vi "Create Scalars for Numeric.vi"() -> ()   [LabVIEW 2021, in "EDT VI Script.lvlib"]
uses:
  Numeric Representation to Type Cast.ctl
  <vilib>/numeric/LVNumericRepresentation.ctl
  EDT VI Script.lvlib
panel:
  in  "Template VI Path":path=path "C:/Users/OneEd/OneDrive/Documents/LabVIEW/edt.lib/numeric.lib/Random in Range (Double).vi"
  in  "PlaceHolders":string[](array[string])=["hi", "lo", "random"]
  out "Slide":dbl(slide) scale=0.0..1.0
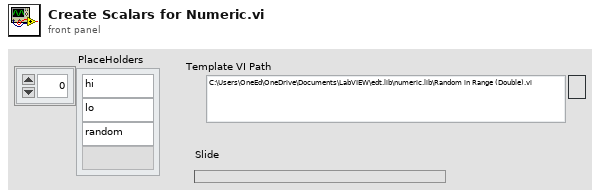
[diagram p1: front panel]
types:
  T1 = typedef "EDT VI Script.lvlib/Numeric Representation to Type Cast.ctl" = map{T2, i32}
  T2 = typedef "LVNumericRepresentation.ctl" = enum32{"Extended Precision", "Double Precision", "Single Precision", "Long", "Word", "Byte", "Unsigned Long", "Unsigned Word", "Unsigned Byte", "Complex Extended", "Complex Double", "Complex Single", "Quad", "Unsigned Quad", "Fixed-Point"}
  T3 = cluster{"Placeholder Name":string, "Function Type":i32}
  T4 = cluster{"Placeholder Name":string, "Numeric Representation":T2}
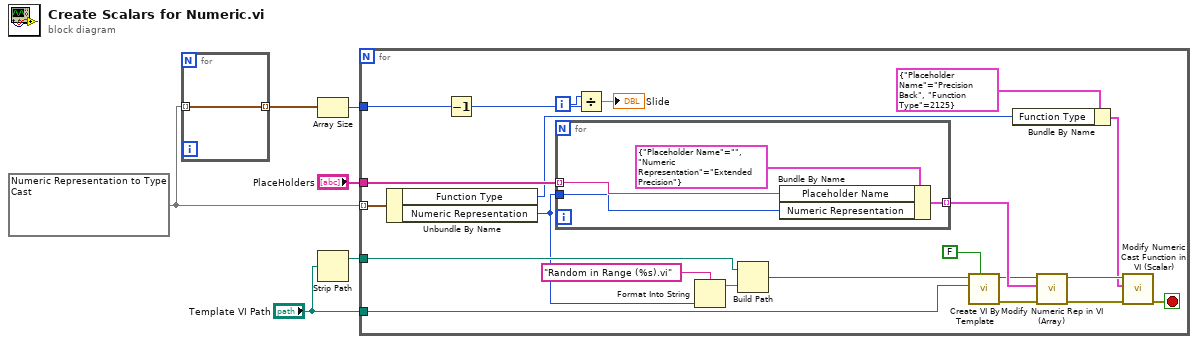
[diagram p0: block diagram]
diagram:
  w2 = T1 {enum."Extended Precision"=1154, enum."Double Precision"=1152, enum."Single Precision"=1151, enum."Long"=1142, enum."Word"=1141, enum."Byte"=1140, enum."Unsigned Long"=1145, enum."Unsigned Word"=1144, enum."Unsigned Byte"=1143, enum."Quad"=1155, enum."Unsigned Quad"=1156, enum."Fixed-Point"=5561} ("SQLite Data Type to LV Data Type")
  n1 = for {
    tunnel: [w7] -> w1 mode=indexing
    tunnel: w2 -> [w7] mode=indexing
  }
  n2 = Array Size(array=w1) -> (size(s)=w6:i32)
  n3 = Strip Path(path="Template VI Path") -> (stripped path=w3:path)  [unwired: 1 out]
  n4 = for {
    tunnel: w6 -> [w27]
    tunnel: "PlaceHolders" -> [w24]
    tunnel: "Template VI Path" -> [w21]
    tunnel: w3 -> [w23]
    tunnel: w2 -> [w18] mode=indexing
    i -> [w26]
    stop <- w19 stop-if-true
    n5 = Unbundle By Name(w18) -> ("Function Type"=w11:i32, "Numeric Representation"=w10:T2)
    n6 = Decrement(x=w27) -> (x-1=w9:i32)
    n7 = for {
      tunnel: w24 -> [w32] mode=indexing
      tunnel: w10 -> [w30]
      tunnel: [w31] -> w22 mode=indexing
      n8 = Bundle By Name(cluster=T4 {"Placeholder Name"="", "Numeric Representation"=enum."Extended Precision"} ("Modify Numeric Representation Param"), "Placeholder Name"=w32, "Numeric Representation"=w30) -> (w31:T4)
    }
    n9 = Divide(x=w26, y=w9) -> (x/y=→"Slide":dbl)
    n10 = Format Into String(format string="Random in Range (%s).vi", w10) -> (resulting string=w28:string)  [unwired: 2 in, 1 out]
    n11 = Build Path(base path=w23, name or relative path=w28) -> (appended path=w20:path)
    n12 = call "Create VI By Template.vi"("Modify Icon?"=FALSE, "Template VI Path"=w21, "Save as"=w20) -> ("error out"=w14:errorcluster, "Save as out"=w13:path)  [unwired: 7 in]
    n13 = Bundle By Name(cluster=T3 {"Placeholder Name"="Precision Back", "Function Type"=2125} ("Modify Numeric Representation Param"), "Function Type"=w11) -> (w12:T3)
    n14 = call "Modify Numeric Rep in VI (Array).vi"("error in"=w14, "Numeric Representation Param"=w22, "Original VI"=w13) -> ("error out"=w15:errorcluster, "Save as out"=w16:path)  [unwired: 7 in]
    n15 = call "Modify Numeric Cast Function in VI (Scalar).vi"("error in"=w15, "Modify Numeric Representation Param"=w12, "Original VI"=w16) -> ("error out"=w19:errorcluster)  [unwired: 7 in, 1 out]
  }
